vi "clLabview_readVI.vi"(11 "vi_lib.lvlib:clFileReader.lvclass":refnum<class "clFileReader.lvclass">) -> (3 "vi_lib.lvlib:clLabview.lvclass 2":refnum<class "clLabview.lvclass">)   [LabVIEW 2011, in "vi_lib.lvlib" / "clLabview.lvclass"]
uses:
  clLabview.lvclass
  clFileReader/clFileReader.lvclass
  clLabview.lvclass/clLabview.ctl
panel:
  in  "vi_lib.lvlib:clLabview.lvclass":refnum<class "clLabview.lvclass">
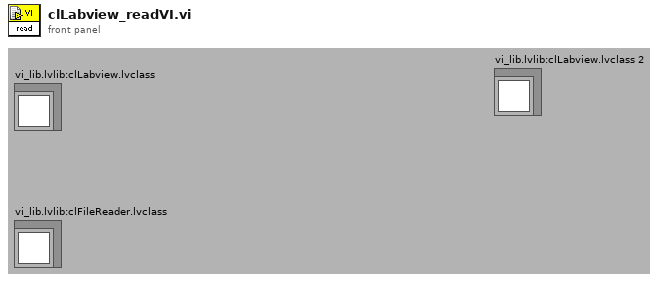
[diagram p1: front panel]
types:
  T1 = cluster{"BlockInfoOffset":u32, "BlockCount":u32, "BlockName":string, "INT2":u32, "INT3":u32, "INT1":u32, "BlockOffset":u32, "INT4":u32, "BlockFileSize":u32}[]
  T2 = cluster{"BlockInfoOffset":u32, "BlockCount":u32, "BlockName":string, "INT2":u32, "INT3":u32, "INT1":u32, "BlockOffset":u32, "INT4":u32, "BlockFileSize":u32}
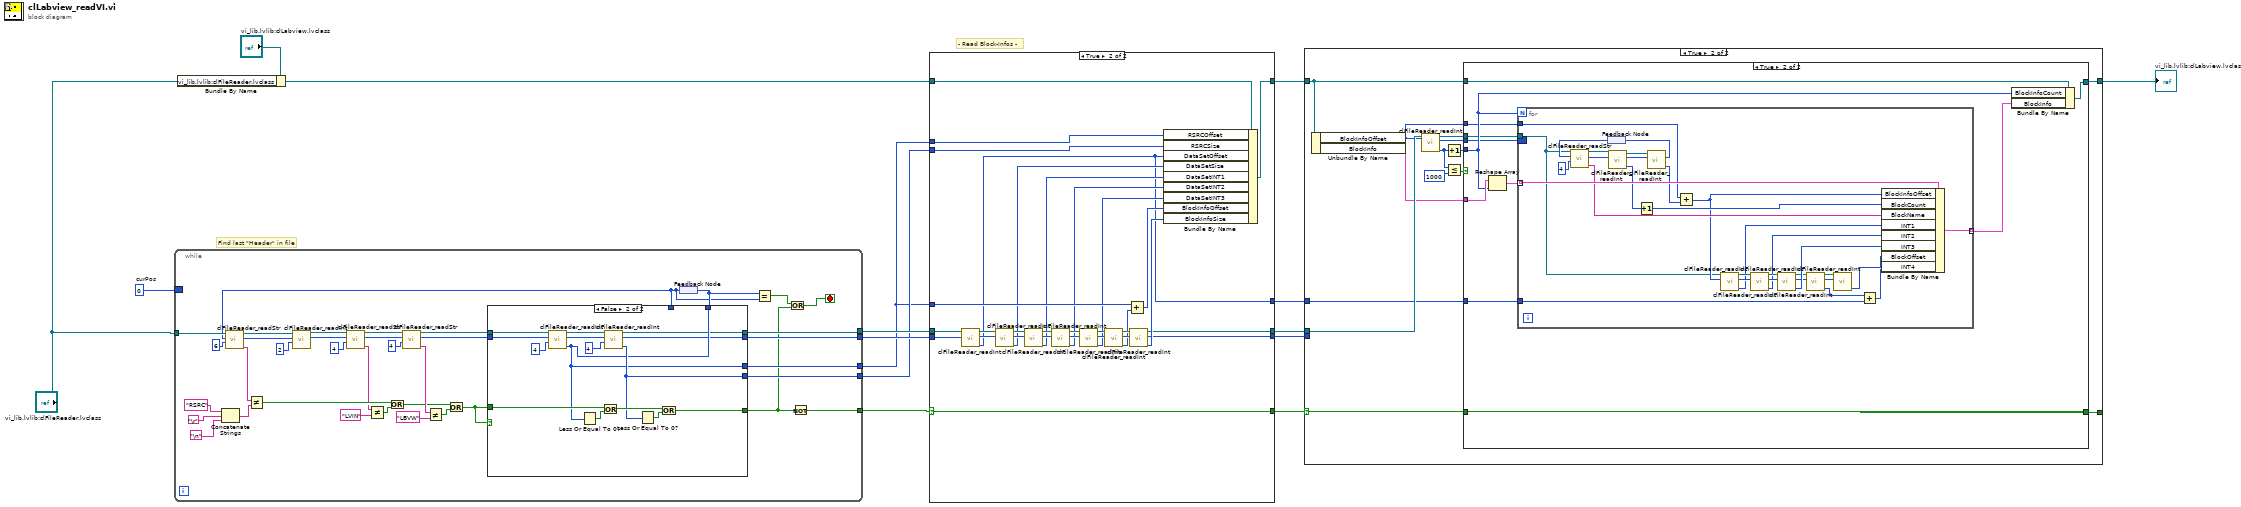
[diagram p0: block diagram]
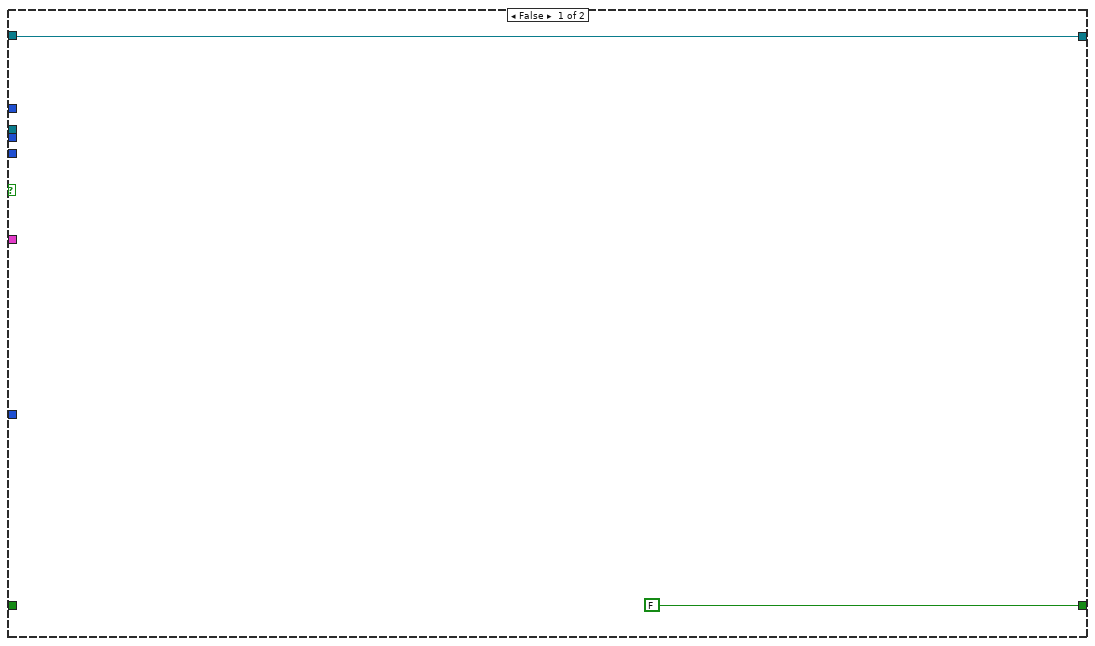
[diagram p3: hidden frame]
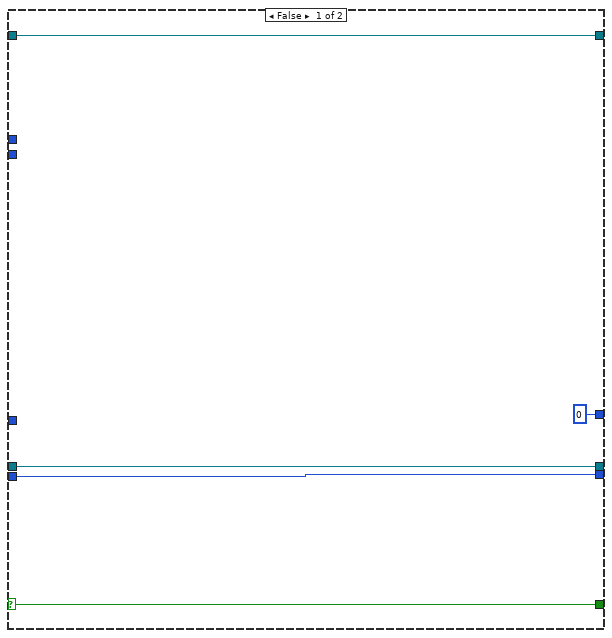
[diagram p4: hidden frame]
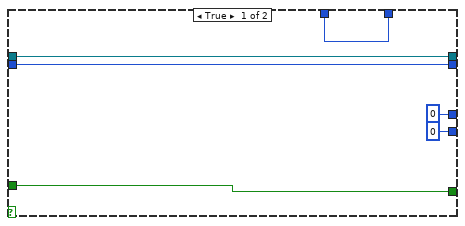
[diagram p5: hidden frame]
diagram:
  w15 = 0  # curPos
  # "- Read Block-Infos -"
  # "Find last \"Header\" in file"
  n1 = while {
    tunnel: "vi_lib.lvlib:clFileReader.lvclass" -> [w52]
    tunnel: [w24] -> w8
    border: w15 -> [_]
    tunnel: [w23] -> w7
    tunnel: [w22] -> w14
    tunnel: [w21] -> w13
    tunnel: [w18] -> w12
    stop <- w25 stop-if-true
    n2 = Concatenate Strings("RSRC" ("y"), "\r", "\n") -> (w37:string)
    n3 = feedback #1() -> (w19:u32)
    n4 = call "clFileReader_readStr.vi"("size"=u32 6, "offset"=w19, "clFileReader.lvclass IN"=w52) -> ("ReadStr - OUT Value"=w41:string, "new offset"=w49:u32, "clFileReader.lvclass OUT"=w50:refnum<class "clFileReader.lvclass">)  [unwired: 6 out]
    n5 = Not Equal?(x=w41, y=w37) -> (x != y?=w36:bool)
    n6 = call "clFileReader_readInt.vi"("size"=u32 2, "offset"=w49, "clFileReader.lvclass IN"=w50) -> ("new offset"=w47:u32, "clFileReader.lvclass OUT"=w46:refnum<class "clFileReader.lvclass">)  [unwired: 7 out]
    n7 = call "clFileReader_readStr.vi"("size"=u32 4, "offset"=w47, "clFileReader.lvclass IN"=w46) -> ("ReadStr - OUT Value"=w34:string, "new offset"=w44:u32, "clFileReader.lvclass OUT"=w45:refnum<class "clFileReader.lvclass">)  [unwired: 6 out]
    n8 = Not Equal?(x=w34, y="LVIN") -> (x != y?=w35:bool)
    n9 = Or(x=w36, y=w35) -> (x .or. y?=w29:bool)
    n10 = call "clFileReader_readStr.vi"("size"=u32 4, "offset"=w44, "clFileReader.lvclass IN"=w45) -> ("ReadStr - OUT Value"=w30:string, "new offset"=w27:u32, "clFileReader.lvclass OUT"=w28:refnum<class "clFileReader.lvclass">)  [unwired: 6 out]
    n11 = Not Equal?(x=w30, y="LBVW") -> (x != y?=w32:bool)
    n12 = Or(x=w29, y=w32) -> (x .or. y?=w26:bool)
    n13 = case shown="False" w26 {
      tunnel: w28 -> [w54 w69]
      tunnel: w27 -> [w53 w70]
      tunnel: w26 -> [w58 w68]
      tunnel: [w58 w64] -> w16
      tunnel: [w57 w62] -> w20
      tunnel: w19 -> [w57 _]
      tunnel: [u32 0 ("OUT Value") w63] -> w24
      tunnel: [u32 0 ("OUT Value") w62] -> w23
      tunnel: [w54 w61] -> w22
      tunnel: [w53 w60] -> w21
      frame True {
      }
      frame False {
        n14 = call "clFileReader_readInt.vi"("size"=u32 4, "offset"=w70, "clFileReader.lvclass IN"=w69) -> ("OUT Value"=w62:u32, "new offset"=w59:u32)  [unwired: 7 out]
        n15 = Less Or Equal To 0?(x=w62) -> (x <= 0?=w67:bool)
        n16 = Or(x=w68, y=w67) -> (x .or. y?=w65:bool)
        n17 = call "clFileReader_readInt.vi"("size"=u32 4, "offset"=w59, "clFileReader.lvclass IN"=w69) -> ("OUT Value"=w63:u32, "new offset"=w60:u32, "clFileReader.lvclass OUT"=w61:refnum<class "clFileReader.lvclass">)  [unwired: 6 out]
        n18 = Less Or Equal To 0?(x=w63) -> (x <= 0?=w66:bool)
        n19 = Or(x=w65, y=w66) -> (x .or. y?=w64:bool)
      }
    }
    n20 = feedback-in #1(w20) -> ()
    n21 = Equal?(x=w20, y=w19) -> (x = y?=w17:bool)
    n22 = Or(x=w17, y=w16) -> (x .or. y?=w25:bool)
    n23 = Not(x=w16) -> (.not. x?=w18:bool)
  }
  n24 = Bundle By Name(cluster="vi_lib.lvlib:clLabview.lvclass", "vi_lib.lvlib:clFileReader.lvclass"="vi_lib.lvlib:clFileReader.lvclass") -> (w9:refnum<class "clLabview.lvclass">)
  n25 = case shown="True" w12 {
    selector: w12 -> [w77 w91]
    tunnel: w14 -> [w75 w107]
    tunnel: w13 -> [w74 w106]
    tunnel: w7 -> [_ w92]
    tunnel: [w77 w91] -> w4
    tunnel: w9 -> [w76 w90]
    tunnel: [w76 w89] -> w6
    tunnel: w8 -> [_ w83]
    tunnel: w7 -> [_ w82]
    tunnel: [w75 w81] -> w3
    tunnel: [w74 w80] -> w2
    tunnel: [u32 0 ("OUT Value") w78] -> w1
    frame False {
    }
    frame True {
      n26 = call "clFileReader_readInt.vi"("offset"=w106, "clFileReader.lvclass IN"=w107) -> ("OUT Value"=w78:u32, "new offset"=w104:u32, "clFileReader.lvclass OUT"=w105:refnum<class "clFileReader.lvclass">)  [unwired: 1 in, 6 out]
      n27 = call "clFileReader_readInt.vi"("offset"=w104, "clFileReader.lvclass IN"=w105) -> ("OUT Value"=w79:u32, "new offset"=w100:u32, "clFileReader.lvclass OUT"=w103:refnum<class "clFileReader.lvclass">)  [unwired: 1 in, 6 out]
      n28 = call "clFileReader_readInt.vi"("offset"=w100, "clFileReader.lvclass IN"=w103) -> ("OUT Value"=w84:u32, "new offset"=w101:u32, "clFileReader.lvclass OUT"=w102:refnum<class "clFileReader.lvclass">)  [unwired: 1 in, 6 out]
      n29 = call "clFileReader_readInt.vi"("offset"=w101, "clFileReader.lvclass IN"=w102) -> ("OUT Value"=w85:u32, "new offset"=w98:u32, "clFileReader.lvclass OUT"=w99:refnum<class "clFileReader.lvclass">)  [unwired: 1 in, 6 out]
      n30 = call "clFileReader_readInt.vi"("offset"=w98, "clFileReader.lvclass IN"=w99) -> ("OUT Value"=w86:u32, "new offset"=w96:u32, "clFileReader.lvclass OUT"=w97:refnum<class "clFileReader.lvclass">)  [unwired: 1 in, 6 out]
      n31 = call "clFileReader_readInt.vi"("offset"=w96, "clFileReader.lvclass IN"=w97) -> ("OUT Value"=w93:u32, "new offset"=w94:u32, "clFileReader.lvclass OUT"=w95:refnum<class "clFileReader.lvclass">)  [unwired: 1 in, 6 out]
      n32 = Add(x=w92, y=w93) -> (x+y=w87:u32)
      n33 = call "clFileReader_readInt.vi"("offset"=w94, "clFileReader.lvclass IN"=w95) -> ("OUT Value"=w88:u32, "new offset"=w80:u32, "clFileReader.lvclass OUT"=w81:refnum<class "clFileReader.lvclass">)  [unwired: 1 in, 6 out]
      n34 = Bundle By Name(cluster=w90, "RSRCOffset"=w82, "RSRCSize"=w83, "DataSetOffset"=w78, "DataSetSize"=w79, "DataSetINT1"=w84, "DataSetINT2"=w85, "DataSetINT3"=w86, "BlockInfoOffset"=w87, "BlockInfoSize"=w88) -> (w89:refnum<class "clLabview.lvclass">)
    }
  }
  n35 = case shown="True" w4 {
    selector: w4 -> [w108 w114]
    tunnel: w6 -> [w109 w123]
    tunnel: [w109 w122] -> w5
    tunnel: w3 -> [_ w121]
    tunnel: w2 -> [_ _]
    tunnel: [w108 w113] -> _
    tunnel: w1 -> [_ w110]
    frame False {
    }
    frame True {
      n36 = Unbundle By Name(w123) -> ("BlockInfoOffset"=w115:u32, "BlockInfo"=w118:T1)
      n37 = call "clFileReader_readInt.vi"("offset"=w115, "clFileReader.lvclass IN"=w121) -> ("OUT Value"=w112:u32, "new offset"=w117:u32, "clFileReader.lvclass OUT"=w116:refnum<class "clFileReader.lvclass">)  [unwired: 1 in, 6 out]
      n38 = Increment(x=w112) -> (x+1=w111:u32)
      n39 = Less Or Equal?(x=w112, y=u32 1000) -> (x <= y?=w119:bool)
      n40 = case shown="True" w119 {
        tunnel: w123 -> [w125 w136]
        tunnel: [w125 w135] -> w122
        tunnel: w111 -> [_ w133]
        tunnel: w118 -> [_ w134]
        tunnel: w117 -> [_ w130]
        tunnel: w116 -> [_ w129]
        tunnel: w115 -> [_ w128]
        tunnel: w114 -> [_ w127]
        tunnel: [FALSE w127] -> w113
        tunnel: w110 -> [_ w126]
        frame False {
        }
        frame True {
          n41 = Reshape Array(w134, w133) -> (w132:T1)
          n42 = for {
            N: w133 -> [_]
            tunnel: w132 -> [w167] mode=indexing
            tunnel: [w166] -> w131 mode=indexing
            tunnel: w129 -> [w152]
            tunnel: w128 -> [w156]
            border: w130 -> [_]
            tunnel: w126 -> [w139]
            n43 = feedback #2() -> (w164:u32)
            n44 = call "clFileReader_readStr.vi"("size"=u32 4, "offset"=w164, "clFileReader.lvclass IN"=w152) -> ("ReadStr - OUT Value"=w165:string, "new offset"=w161:u32, "clFileReader.lvclass OUT"=w162:refnum<class "clFileReader.lvclass">)  [unwired: 6 out]
            n45 = call "clFileReader_readInt.vi"("offset"=w161, "clFileReader.lvclass IN"=w162) -> ("OUT Value"=w160:u32, "new offset"=w157:u32, "clFileReader.lvclass OUT"=w158:refnum<class "clFileReader.lvclass">)  [unwired: 1 in, 6 out]
            n46 = Increment(x=w160) -> (x+1=w159:u32)
            n47 = call "clFileReader_readInt.vi"("offset"=w157, "clFileReader.lvclass IN"=w158) -> ("OUT Value"=w155:u32, "new offset"=w154:u32)  [unwired: 1 in, 7 out]
            n48 = feedback-in #2(w154) -> ()
            n49 = Add(x=w156, y=w155) -> (x+y=w153:u32)
            n50 = call "clFileReader_readInt.vi"("offset"=w153, "clFileReader.lvclass IN"=w152) -> ("OUT Value"=w147:u32, "new offset"=w150:u32, "clFileReader.lvclass OUT"=w151:refnum<class "clFileReader.lvclass">)  [unwired: 1 in, 6 out]
            n51 = call "clFileReader_readInt.vi"("offset"=w150, "clFileReader.lvclass IN"=w151) -> ("OUT Value"=w146:u32, "new offset"=w148:u32, "clFileReader.lvclass OUT"=w149:refnum<class "clFileReader.lvclass">)  [unwired: 1 in, 6 out]
            n52 = call "clFileReader_readInt.vi"("offset"=w148, "clFileReader.lvclass IN"=w149) -> ("OUT Value"=w145:u32, "new offset"=w144:u32, "clFileReader.lvclass OUT"=w140:refnum<class "clFileReader.lvclass">)  [unwired: 1 in, 6 out]
            n53 = call "clFileReader_readInt.vi"("offset"=w144, "clFileReader.lvclass IN"=w140) -> ("OUT Value"=w138:u32, "new offset"=w142:u32, "clFileReader.lvclass OUT"=w143:refnum<class "clFileReader.lvclass">)  [unwired: 1 in, 6 out]
            n54 = call "clFileReader_readInt.vi"("offset"=w142, "clFileReader.lvclass IN"=w143) -> ("OUT Value"=w141:u32)  [unwired: 1 in, 8 out]
            n55 = Add(x=w138, y=w139) -> (x+y=w137:u32)
            n56 = Bundle By Name(cluster=w167, "BlockInfoOffset"=w153, "BlockCount"=w159, "BlockName"=w165, "INT1"=w147, "INT2"=w146, "INT3"=w145, "BlockOffset"=w137, "INT4"=w141) -> (w166:T2)
          }
          n57 = Bundle By Name(cluster=w136, "BlockInfoCount"=w133, "BlockInfo"=w131) -> (w135:refnum<class "clLabview.lvclass">)
        }
      }
    }
  }
  "vi_lib.lvlib:clLabview.lvclass 2" <- w5
